vi "Delete Item.vi"(8 "error in (no error)":errorcluster, 11 "PLC_Module in":refnum<class "PLC_Module.lvclass">) -> (0 "error out":errorcluster, 3 "PLC_Module out":refnum<class "PLC_Module.lvclass">)   [LabVIEW 2025, in "PLC_Module.lvlib" / "PLC_Module.lvclass"]
uses:
  PLC_Module.lvclass
  PLC_Module.lvclass/PLC_Module.ctl
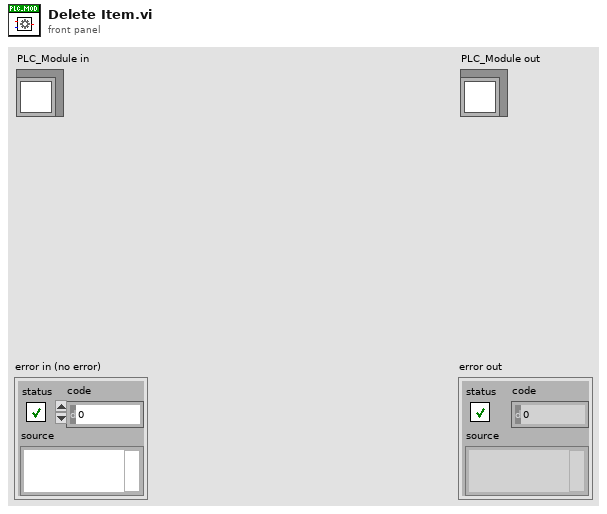
[diagram p1: front panel]
types:
  T1 = typedef "PLC_Module.lvlib/PLC_Module.lvclass/PLC_Data_Config.ctl" = map{string, cluster{"Config":T2, "Get Value":string, "Set Value":string}}
  T2 = typedef "PLC_Module.lvlib/PLC_Module.lvclass/PLC_Data.ctl" = cluster{"Address":string, "Direction":enum16{"PC->PLC", "PLC->PC"}, "DataType":T3, "Description":string}
  T3 = typedef "PLC_Module.lvlib/PLC_Module.lvclass/PLC_Data_Type.ctl" = enum16{"Boolean", "Single Float", "U8", "U32", "U32_Array", "String"}
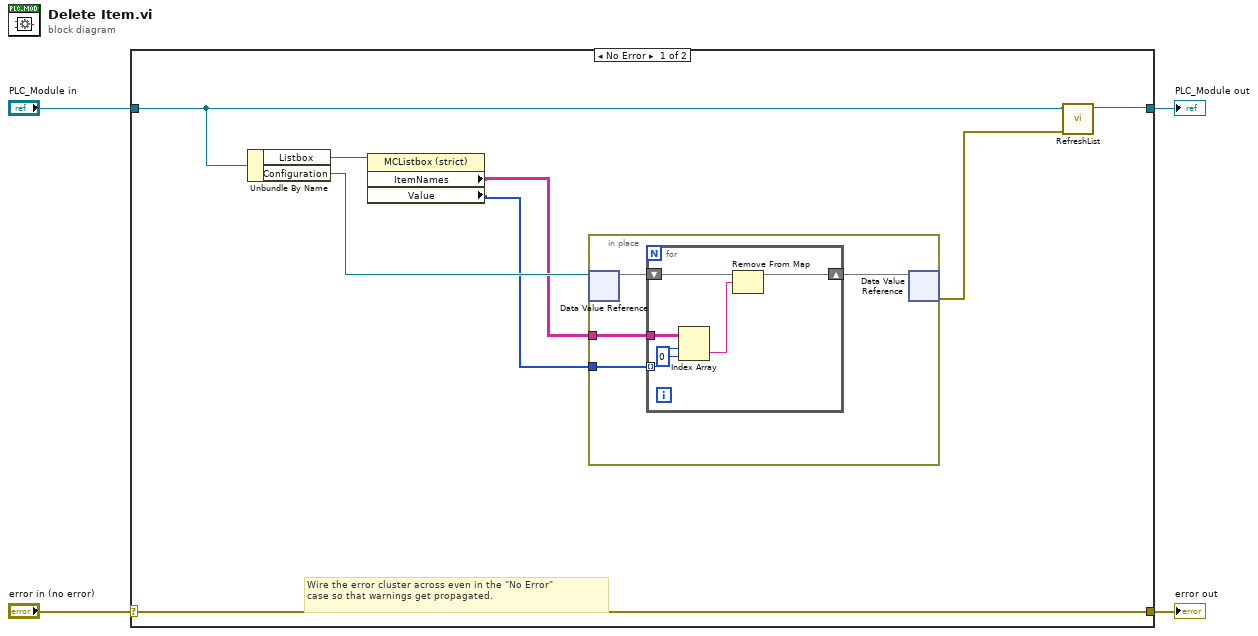
[diagram p0: block diagram]
diagram:
  n1 = case shown="No Error" "error in (no error)" {
    selector: "error in (no error)" -> [w12 w24]
    tunnel: [w12 w24] -> w3
    tunnel: [w8 w23] -> w1
    tunnel: "PLC_Module in" -> [w9 w23]
    frame No Error {
      # "Wire the error cluster across even in the \"No Error\"\ncase so that warnings get propagated."
      n2 = Unbundle By Name(w9) -> ("Listbox"=w11:refnum<vi>, "Configuration"=w10:refnum<data-value>)
      n3 = property class="MCListbox (strict)"(reference=w11) -> ("ItemNames"=w5:string[][], "Value"=w6:i32[])  [unwired: 1 in, 2 out]
      n4 = in-place {
        in-place-border: w6 -> [w14]
        in-place-border: w5 -> [w13]
        n5 = in-place-dvr #1(w10) -> (w16:T1)  [unwired: 1 out]
        n6 = for {
          shift-right: [w21] -> w15
          shift-left: w16 -> [w22]
          tunnel: w14 -> [w20] mode=indexing
          tunnel: w13 -> [w19]
          n7 = Index Array(array=w19, index (row)=w20, index (col)=0 ("disabled index (col)")) -> (element=w17:string)
          n8 = Remove From Map(10:w17, 11:w22) -> (3:w21:T1)  [unwired: 2 out]
        }
        n9 = in-place-dvr #1(w15) -> (w7:errorcluster)  [unwired: 1 out]
      }
      n10 = call "RefreshList.vi"("error in (no error)"=w7, "PLC_Module in"=w9) -> ("PLC_Module out"=w8:refnum<class "PLC_Module.lvclass">)  [unwired: 8 in, 1 out]
    }
    frame Error {
    }
  }
  "error out" <- w3
  "PLC_Module out" <- w1
